vi "Thermopower-v2-SMU1norangespec.vi"(0 "Gate Start":dbl format="%#_13g", 1 "hold time (sec)":dbl=10.0 format="%#_13g", 2 "Gate step - extra milliseconds to wait":u32=20000, 4 "N Gate Intervals":i32=7, 5 "Gate Step":dbl=-6.0, 6 "N Heater Intervals":i32=7, 7 "Heater Step":dbl=3.3) -> ()   [LabVIEW 2016]
uses:
  <vilib>/Utility/file.llb/Write To Spreadsheet File (DBL).vi
  <vilib>/Utility/file.llb/Read From Spreadsheet File (DBL).vi
  Driver/New driver/Agilent 415X Series.lvlib
panel:
  out "Voltage across heater (VSU 1 and SMU4) 2":dbl[][](graph)
  out "error out 2":errorcluster
  out "Gate Voltage (SMU 3) 2":dbl[](graph)
  out "Thermal Voltage (SMU2), SMU1 is Common 2":dbl[](graph)
  out "SPA VISA resource name 2":refnum<visa-resource-name>
  out "Voltage across heater (VSU 1 and SMU4)":dbl[][](graph)
  out "Gate Voltage (SMU 3)":dbl[](graph)
  out "Thermal Voltage (SMU2), SMU1 is Common":dbl[](graph)
  in  "SPA VISA resource name":refnum<visa-resource-name>="GPIB0::14::INSTR"
  in  "error in (no error)":errorcluster
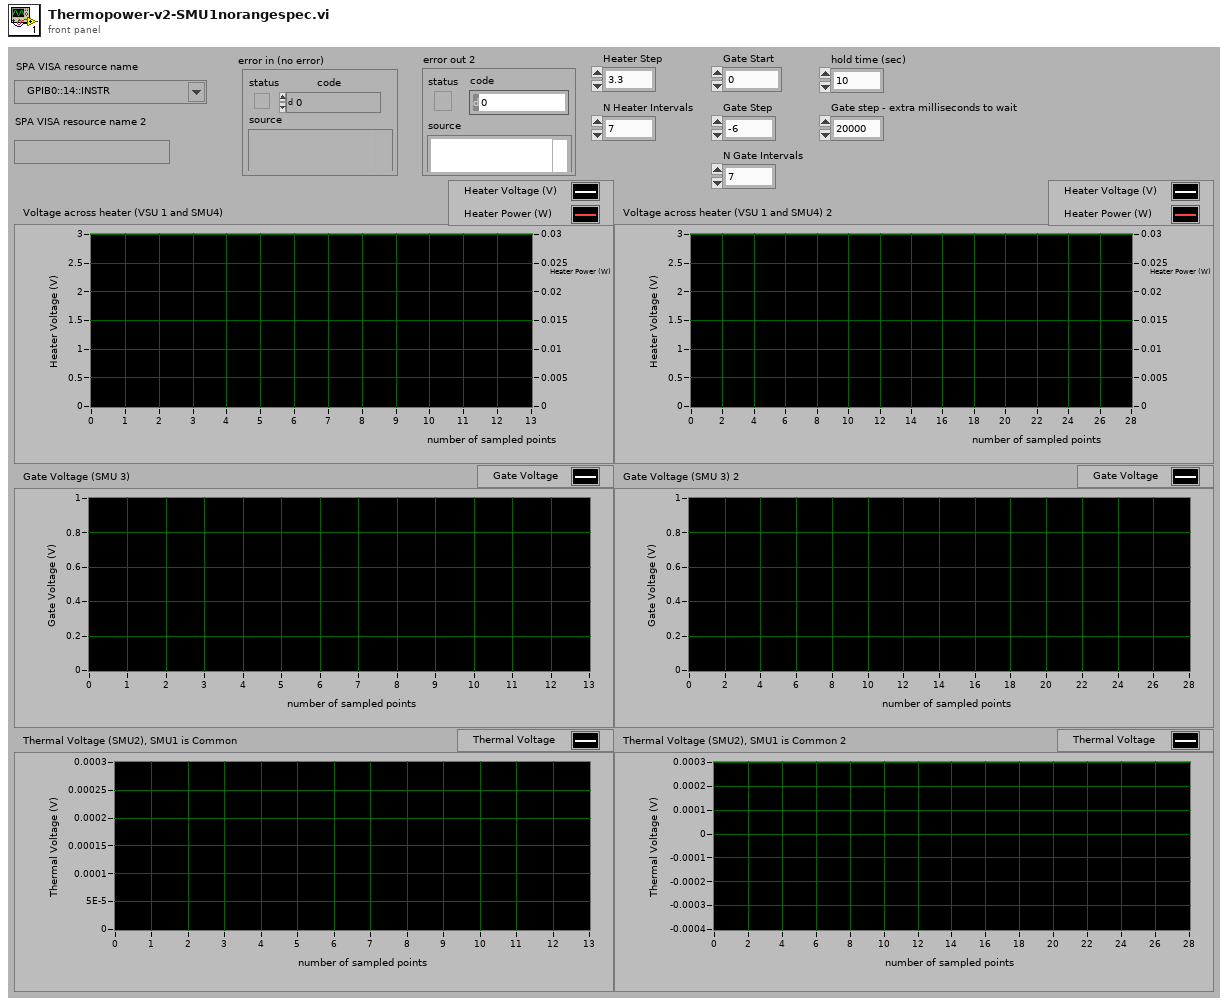
[diagram p1: front panel]
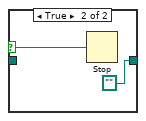
[diagram p3: hidden frame]
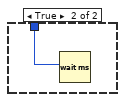
[diagram p4: hidden frame]
diagram:
  # "calculate end gate voltage"
  n1 = flat-sequence {
    tunnel: "error in (no error)" -> [w51]
    tunnel: "SPA VISA resource name" -> [w50]
    tunnel: [w49] -> w45
    tunnel: [w48] -> w44
    tunnel: w45 -> [w58]
    tunnel: w44 -> [w57]
    tunnel: [w54] -> w43
    tunnel: [w53] -> w42
    tunnel: w43 -> [w66]
    tunnel: w42 -> [w65]
    tunnel: [w64] -> w41
    tunnel: [w63] -> w40
    tunnel: w41 -> [w77]
    tunnel: w40 -> [w76]
    tunnel: [w75] -> w39
    tunnel: [w74] -> w38
    tunnel: w39 -> [w88]
    tunnel: w38 -> [w87]
    tunnel: [w86] -> w37
    tunnel: [w85] -> w35
    tunnel: w37 -> [w93]
    tunnel: [w94] -> w36
    tunnel: w35 -> [w92]
    tunnel: [w95] -> w34
    tunnel: w36 -> [w110]
    tunnel: w34 -> [w112]
    tunnel: [w111] -> w27
    tunnel: [w109] -> w26
    tunnel: w27 -> [w114]
    tunnel: w26 -> [w113]
    tunnel: [w117] -> w2
    tunnel: [w116] -> w1
    tunnel: [w127] -> w33
    tunnel: [w130] -> w32
    tunnel: [w129] -> w5
    tunnel: w2 -> [w127]
    tunnel: w1 -> [w128]
    frame #0 {
      n2 = call "Initialize.vi"("error in (no error)"=w51, "reset"=TRUE, "VISA resource name"=w50) -> ("error out"=w48:errorcluster, "VISA resource name out"=w49:refnum<visa-resource-name>)  [unwired: 2 in, 5 out]
    }
    frame #1 {
      n3 = call "Select-Meas. Mode.vi"("clear all channels"=TRUE, "error in (no error)"=w57, "measurement mode"=TRUE, "VISA resource name"=w58) -> ("error out"=w53:errorcluster, "VISA resource name out"=w54:refnum<visa-resource-name>)  [unwired: 1 in, 5 out]
    }
    frame #2 {
      w61 = 0 items=["0  ", "10K Ohms  ", "100K Ohms  ", "1M Ohms  "] ("series resistance *")
      w62 = 2 items=["V  ", "I  ", "  common  "] ("mode")
      w67 = 0 items=["SMU1  ", "SMU2  ", "SMU3  ", "SMU4  ", "SMU5  ", "SMU6  "] ("unit to configure")
      # "SMU1 configured to be common"
      n4 = call "Config-Chan-SMU-Sampling.vi"("VISA resource name in"=w66, "function"=TRUE, "series resistance *"=w61, "unit to configure"=w67, "V name (max 6 chars)"="Vgnd", "standby"=TRUE, "error in (no error)"=w65, "mode"=w62, "I name (max 6 chars)"="Ignd") -> ("VISA resource name out"=w64:refnum<visa-resource-name>, "error out"=w63:errorcluster)  [unwired: 5 out]
    }
    frame #3 {
      w71 = 0 items=["0  ", "10K Ohms  ", "100K Ohms  ", "1M Ohms  "] ("series resistance *")
      w73 = 1 items=["V  ", "I  ", "  common  "] ("mode")
      w78 = 1 items=["SMU1  ", "SMU2  ", "SMU3  ", "SMU4  ", "SMU5  ", "SMU6  "] ("unit to configure")
      # "SMU2 configured to source current (to be set to zero) \nand measure the thermal voltage"
      n5 = call "Config-Chan-SMU-Sampling.vi"("VISA resource name in"=w77, "function"=TRUE, "series resistance *"=w71, "unit to configure"=w78, "V name (max 6 chars)"="Vth", "standby"=TRUE, "error in (no error)"=w76, "mode"=w73, "I name (max 6 chars)"="Ith") -> ("VISA resource name out"=w75:refnum<visa-resource-name>, "error out"=w74:errorcluster)  [unwired: 5 out]
    }
    frame #4 {
      w82 = 0 items=["0  ", "10K Ohms  ", "100K Ohms  ", "1M Ohms  "] ("series resistance *")
      w84 = 0 items=["V  ", "I  ", "  common  "] ("mode")
      w89 = 2 items=["SMU1  ", "SMU2  ", "SMU3  ", "SMU4  ", "SMU5  ", "SMU6  "] ("unit to configure")
      # "SMU3 configured to source a gate voltage"
      n6 = call "Config-Chan-SMU-Sampling.vi"("VISA resource name in"=w88, "function"=TRUE, "series resistance *"=w82, "unit to configure"=w89, "V name (max 6 chars)"="Vg", "standby"=TRUE, "error in (no error)"=w87, "mode"=w84, "I name (max 6 chars)"="Ig") -> ("VISA resource name out"=w86:refnum<visa-resource-name>, "error out"=w85:errorcluster)  [unwired: 5 out]
    }
    frame #5 {
      w97 = 0 items=["0  ", "10K Ohms  ", "100K Ohms  ", "1M Ohms  "] ("series resistance *")
      w99 = 2 items=["V  ", "I  ", "  common  "] ("mode")
      w100 = 3 items=["SMU1  ", "SMU2  ", "SMU3  ", "SMU4  ", "SMU5  ", "SMU6  "] ("unit to configure")
      # "SMU4 configured to heater ground"
      n7 = call "Config-Chan-SMU-Sampling.vi"("VISA resource name in"=w93, "function"=TRUE, "series resistance *"=w97, "unit to configure"=w100, "V name (max 6 chars)"="Vhgnd", "standby"=TRUE, "error in (no error)"=w92, "mode"=w99, "I name (max 6 chars)"="Ihgnd") -> ("VISA resource name out"=w94:refnum<visa-resource-name>, "error out"=w95:errorcluster)  [unwired: 5 out]
    }
    frame #6 {
      # "VSU1 configured to source a voltage accross a heater"
      n8 = call "Config-Chan-VSUs-Sampling.vi"("VISA session"=w110, "VSU1 function"=TRUE, "VSU2 standby"=TRUE, "VSU1 standby"=FALSE, "VSU1 V name \n(max 6 chars)"="VSU1" ("V name (max 6 chars)"), "VSU2 V name \n(max 6 chars)"="VSU2" ("V name (max 6 chars)"), "error in (no error)"=w112, "VSU2 function"=FALSE) -> ("VISA resource name out"=w109:refnum<visa-resource-name>, "error out"=w111:errorcluster)  [unwired: 6 out]
    }
    frame #7 {
      n9 = VISA Write(VISA resource name=w113, write buffer=":PAGE:MEAS:MSET:SMU2:RANG:MODE FIX", error in (no error)=w114) -> (VISA resource name out=w126:refnum<visa-resource-name>, error out=w125:errorcluster)  [unwired: 1 out]
      n10 = VISA Write(VISA resource name=w126, write buffer=":PAGE:MEAS:MSET:SMU2:RANG 2", error in (no error)=w125) -> (VISA resource name out=w121:refnum<visa-resource-name>, error out=w120:errorcluster)  [unwired: 1 out]
      n11 = VISA Write(VISA resource name=w121, write buffer=":PAGE:MEAS:MSET:ITIM LONG", error in (no error)=w120) -> (VISA resource name out=w119:refnum<visa-resource-name>, error out=w118:errorcluster)  [unwired: 1 out]
      n12 = VISA Write(VISA resource name=w119, write buffer=":PAGE:MEAS:MSET:ITIM:LONG 10", error in (no error)=w118) -> (VISA resource name out=w117:refnum<visa-resource-name>, error out=w116:errorcluster)  [unwired: 1 out]
    }
    frame #8 {
      w129 = 0.0 ("source (V or A)")
      w131 = u16 1 items=["SMU 1", "SMU2", "SMU3", "SMU4", "SMU5", "SMU6", "VSU1", "VSU2"] ("unit (SMU1:0)")
      n13 = call "Config-Sampling-Const-Source.vi"("compliance (SMUs only)"=0.0001, "error in (no error)"=w128, "source (V or A)"=w129, "unit (SMU1:0)"=w131, "VISA session"=w127) -> ("error out"=w130:errorcluster)  [unwired: 6 out]
    }
  }
  n14 = Subtract(x="N Gate Intervals", y=1) -> (x-y=w13:i32)
  n15 = Multiply(x=w13, y="Gate Step") -> (x*y=w11:dbl)
  n16 = Add(x=w11, y="Gate Start") -> (x+y=w10:dbl)
  n17 = call "File Dialog"("start path"=path "C:/users old/khk30", "pattern (all files)"="*.txt") -> ("selected path"=w30:path, "cancelled"=w29:bool)  [unwired: 10 in, 2 out]
  n18 = case shown="False" w29 {
    selector: w29 -> [_ w135]
    tunnel: w30 -> [w133 _]
    tunnel: [w133 path ""] -> w17
    frame False {
    }
    frame True {
      n19 = Stop(stop? (T)=w135) -> ()
    }
  }
  n20 = for {
    N: "N Gate Intervals" -> [_]
    tunnel: w17 -> [w147]
    tunnel: w33 -> [w146]
    tunnel: w32 -> [w145]
    tunnel: [w143] -> w21
    tunnel: [w142] -> w20
    tunnel: "N Heater Intervals" -> [w141]
    tunnel: "Gate Step" -> [w140]
    tunnel: "Gate Start" -> [w139]
    tunnel: "Heater Step" -> [w138]
    tunnel: "Gate step - extra milliseconds to wait" -> [w137]
    tunnel: [w136] -> w6 mode=indexing
    i -> [w144]
    n21 = flat-sequence {
      tunnel: w144 -> [w299]
      tunnel: [w304] -> w149
      tunnel: [w303] -> w148
      tunnel: w146 -> [w302]
      tunnel: w145 -> [w301]
      tunnel: w140 -> [w296]
      tunnel: w139 -> [w295]
      frame #0 {
        w305 = u16 2 items=["SMU 1", "SMU2", "SMU3", "SMU4", "SMU5", "SMU6", "VSU1", "VSU2"] ("unit (SMU1:0)")
        n22 = Multiply(x=w296, y=w299) -> (x*y=w298:dbl)
        n23 = Add(x=w295, y=w298) -> (x+y=w297:dbl)
        n24 = call "Config-Sampling-Const-Source.vi"("compliance (SMUs only)"=0.001, "error in (no error)"=w301, "source (V or A)"=w297, "unit (SMU1:0)"=w305, "VISA session"=w302) -> ("error out"=w303:errorcluster, "VISA resource name out"=w304:refnum<visa-resource-name>)  [unwired: 5 out]
      }
    }
    n25 = for {
      N: w141 -> [_]
      tunnel: w149 -> [w168]
      tunnel: w148 -> [w167]
      tunnel: w147 -> [w166]
      tunnel: w144 -> [w159]
      tunnel: [w154] -> w143
      tunnel: [w153] -> w142
      tunnel: w138 -> [w152]
      tunnel: w137 -> [w151]
      tunnel: [w150] -> w136 mode=indexing
      i -> [w169]
      n26 = flat-sequence {
        tunnel: [w186] -> w179
        tunnel: [w185] -> w178
        tunnel: w169 -> [w181]
        tunnel: w168 -> [w184]
        tunnel: w167 -> [w183]
        tunnel: [w181] -> w160
        tunnel: w152 -> [w180]
        tunnel: w179 -> [w196]
        tunnel: w178 -> [w194]
        tunnel: [w195] -> w177
        tunnel: [w194] -> w176
        tunnel: w160 -> [w190]
        tunnel: w159 -> [w189]
        tunnel: w151 -> [w188]
        tunnel: w177 -> [w203]
        tunnel: w176 -> [w202]
        tunnel: [w201] -> w175
        tunnel: [w200] -> w174
        tunnel: ["hold time (sec)"] -> w150
        tunnel: w175 -> [w213]
        tunnel: w174 -> [w212]
        tunnel: [w211] -> w173
        tunnel: [w210] -> w172
        tunnel: w173 -> [w219]
        tunnel: w172 -> [w218]
        tunnel: [w217] -> w171
        tunnel: [w216] -> w170
        tunnel: w171 -> [w238]
        tunnel: w170 -> [w237]
        tunnel: w166 -> [w239]
        tunnel: [w239] -> w165
        tunnel: [w239] -> w164
        tunnel: [w225] -> w162
        tunnel: [w227] -> w154
        tunnel: w165 -> [w266]
        tunnel: [w264] -> w158
        tunnel: w164 -> [w264]
        tunnel: w162 -> [w261]
        tunnel: [w261] -> w156
        tunnel: w158 -> [w270]
        tunnel: [w270] -> w157
        tunnel: w156 -> [w271]
        tunnel: [w271] -> w155
        tunnel: w157 -> [w276]
        tunnel: [w276] -> w163
        tunnel: w155 -> [w272]
        tunnel: [w272] -> w161
        tunnel: w163 -> [w290]
        tunnel: w161 -> [w281]
        tunnel: [w281] -> w153
        frame #0 {
          w187 = u16 6 items=["SMU 1", "SMU2", "SMU3", "SMU4", "SMU5", "SMU6", "VSU1", "VSU2"] ("unit (SMU1:0)")
          n27 = Multiply(x=w180, y=w181) -> (x*y=w182:dbl)
          n28 = call "Config-Sampling-Const-Source.vi"("error in (no error)"=w183, "source (V or A)"=w182, "unit (SMU1:0)"=w187, "VISA session"=w184) -> ("error out"=w186:errorcluster, "VISA resource name out"=w185:refnum<visa-resource-name>)  [unwired: 1 in, 5 out]
        }
        frame #1 {
          n29 = Equal To 0?(x=w190) -> (x = 0?=w191:bool)
          n30 = Greater Than 0?(x=w189) -> (x > 0?=w192:bool)
          n31 = And(x=w191, y=w192) -> (x .and. y?=w193:bool)
          n32 = call "Config-Display-List.vi"("error in (no error)"=w196, "list (max 8 elements)"=string[] ["Vth", "Ith", "VSU1", "Ihgnd", "Vg", "Ig", "Ignd"], "VISA session"=w194) -> ("error out"=w195:errorcluster)  [unwired: 1 in, 7 out]
          n33 = case shown="False" w193 {
            tunnel: w188 -> [_ w198]
            frame False {
            }
            frame True {
              n34 = Wait (ms)(milliseconds to wait=w198) -> ()  [unwired: 1 out]
            }
          }
        }
        frame #2 {
          w204 = 100.0  # sampling time limit
          w205 = 0 items=["linear", "log 10", "log 25", "log 50", "thinned out"] ("mode (linear: 0)")
          w206 = 0 items=["auto (linear only)", "no limit", "set limit "] ("sampling time\n(linear/thinned-out only)")
          w207 = 0.1  # initial interval (sec)
          w208 = 10  # num. of events
          w209 = 1  # number of samples
          n35 = call "Config-Sampling-Parameters.vi"("VISA session"=w202, "mode (linear: 0)"=w205, "initial interval (sec)"=w207, "sampling time\n(linear/thinned-out only)"=w206, "number of samples"=w209, "error in (no error)"=w203, "sampling time limit"=w204, "num. of events"=w208, "hold time (sec)"="hold time (sec)") -> ("VISA resource name out"=w200:refnum<visa-resource-name>, "error out"=w201:errorcluster)  [unwired: 7 in, 10 out]
        }
        frame #3 {
          w215 = 2 items=["short  ", "medium  ", "long  "] ("integration time")
          n36 = call "Config-Meas-Timing.vi"("# PLCs for long integration time"=1, "error in (no error)"=w213, "integration time"=w215, "VISA session"=w212) -> ("error out"=w211:errorcluster, "VISA resource name out"=w210:refnum<visa-resource-name>)  [unwired: 2 in, 4 out]
        }
        frame #4 {
          w221 = 1 items=["stop  ", "single  ", "single-append  ", "stress start  ", "continuous  ", "standby on  ", "standby off  ", "zero  "] ("function (stop:0)")
          n37 = call "Op-Start-Stop.vi"("time to wait (30000ms)"=600000, "error in (no error)"=w219, "function (stop:0)"=w221, "wait until finish"=TRUE, "VISA resource name"=w218) -> ("error out"=w217:errorcluster, "VISA resource name out"=w216:refnum<visa-resource-name>)  [unwired: 5 out]
        }
        frame #5 {
          # "Computes Heater power via P=VI"
          n38 = call "4155C DOWNLOAD variable.vi"("error in (no error)"=w238, "Variable name"="Vth", "VISA resource name in"=w237) -> ("error out"=w246:errorcluster, "Output data"=w233:dbl[], "VISA Resource Name out"=w251:refnum<visa-resource-name>)  [unwired: 2 out]
          n39 = call "4155C DOWNLOAD variable.vi"("error in (no error)"=w246, "Variable name"="Ith", "VISA resource name in"=w251) -> ("error out"=w245:errorcluster, "Output data"=w234:dbl[], "VISA Resource Name out"=w250:refnum<visa-resource-name>)  [unwired: 2 out]
          n40 = call "4155C DOWNLOAD variable.vi"("error in (no error)"=w245, "Variable name"="VSU1", "VISA resource name in"=w250) -> ("error out"=w244:errorcluster, "Output data"=w231:dbl[], "VISA Resource Name out"=w249:refnum<visa-resource-name>)  [unwired: 2 out]
          n41 = call "4155C DOWNLOAD variable.vi"("error in (no error)"=w244, "Variable name"="Ihgnd", "VISA resource name in"=w249) -> ("error out"=w243:errorcluster, "Output data"=w232:dbl[], "VISA Resource Name out"=w248:refnum<visa-resource-name>)  [unwired: 2 out]
          n42 = Multiply(x=w231, y=w232) -> (x*y=w236:dbl[])
          n43 = Absolute Value(x=w236) -> (abs(x)=w230:dbl[])
          n44 = call "4155C DOWNLOAD variable.vi"("error in (no error)"=w243, "Variable name"="Vg", "VISA resource name in"=w248) -> ("error out"=w242:errorcluster, "Output data"=w235:dbl[], "VISA Resource Name out"=w247:refnum<visa-resource-name>)  [unwired: 2 out]
          n45 = call "4155C DOWNLOAD variable.vi"("error in (no error)"=w242, "Variable name"="Ig", "VISA resource name in"=w247) -> ("error out"=w226:errorcluster, "Output data"=w224:dbl[], "VISA Resource Name out"=w229:refnum<visa-resource-name>)  [unwired: 2 out]
          n46 = call "4155C DOWNLOAD variable.vi"("error in (no error)"=w226, "Variable name"="Ignd", "VISA resource name in"=w229) -> ("error out"=w225:errorcluster, "Output data"=w223:dbl[], "VISA Resource Name out"=w227:refnum<visa-resource-name>)  [unwired: 2 out]
          n47 = Build Array(w230, w231, w232, w233, w234, w235, w224, w223) -> (w241:dbl[][])
          n48 = call-poly <vilib>:"Write To Spreadsheet File.vi"("transpose? (no:F)"=TRUE, "format (%.3f)"="%.13f", "append to file? (new file:F)"=TRUE, "2D data"=w241, "file path (dialog if empty)"=w239) -> ()  [unwired: 1 in, 3 out]
        }
        frame #6 {
          # "plot the thermal voltage after reading the file"
          n49 = call-poly <vilib>:"Read From Spreadsheet File.vi"("transpose (no:F)"=TRUE, "format (%.3f)"="%.13f", "max characters/row  (no limit:0)"=0, "number of rows (all:-1)"=-1, "file path (dialog if empty)"=w266) -> ("all rows"=w263:dbl[][])  [unwired: 6 out]
          n50 = Index Array(array=w263, index (row)=3) -> (element=→"Thermal Voltage (SMU2), SMU1 is Common":dbl[])  [unwired: 1 in]
        }
        frame #7 {
        }
        frame #8 {
          # "plot the gate voltage after reading the file"
          n51 = call-poly <vilib>:"Read From Spreadsheet File.vi"("transpose (no:F)"=TRUE, "format (%.3f)"="%.13f", "max characters/row  (no limit:0)"=0, "number of rows (all:-1)"=-1, "file path (dialog if empty)"=w276) -> ("all rows"=w275:dbl[][])  [unwired: 6 out]
          n52 = Index Array(array=w275, index (row)=5) -> (element=→"Gate Voltage (SMU 3)":dbl[])  [unwired: 1 in]
        }
        frame #9 {
          # "plot the voltage across the heater and the \npower dissipated by the heater after reading the file"
          n53 = call-poly <vilib>:"Read From Spreadsheet File.vi"("transpose (no:F)"=TRUE, "format (%.3f)"="%.13f", "max characters/row  (no limit:0)"=0, "number of rows (all:-1)"=-1, "file path (dialog if empty)"=w290) -> ("all rows"=w288:dbl[][])  [unwired: 6 out]
          n54 = Index Array(array=w288, index (row)=1) -> (element=w282:dbl[])  [unwired: 1 in]
          n55 = Index Array(array=w288, index (row)=2) -> (element=w286:dbl[])  [unwired: 1 in]
          n56 = Multiply(x=w282, y=w286) -> (x*y=w285:dbl[])
          n57 = Absolute Value(x=w285) -> (abs(x)=w284:dbl[])
          n58 = Build Array(w282, w284) -> (→"Voltage across heater (VSU 1 and SMU4)":dbl[][])
        }
      }
    }
  }
  n59 = flat-sequence {
    tunnel: [w313] -> w25
    tunnel: [w312] -> w24
    tunnel: w21 -> [w307]
    tunnel: w20 -> [w306]
    tunnel: w25 -> [w324]
    tunnel: w24 -> [w323]
    tunnel: [w318] -> w4
    tunnel: [w317] -> w3
    tunnel: [w328] -> w23
    tunnel: [w329] -> w22
    tunnel: w4 -> [w331]
    tunnel: w3 -> [w330]
    tunnel: w23 -> [w339]
    tunnel: w22 -> [w340]
    tunnel: [w338] -> w18
    tunnel: [w337] -> w19
    tunnel: w5 -> [w336]
    frame #0 {
      w310 = 0 items=["0  ", "10K Ohms  ", "100K Ohms  ", "1M Ohms  "] ("series resistance *")
      w311 = 2 items=["V  ", "I  ", "  common  "] ("mode")
      w314 = 1 items=["SMU1  ", "SMU2  ", "SMU3  ", "SMU4  ", "SMU5  ", "SMU6  "] ("unit to configure")
      # "SMU2 configured to be common"
      n60 = call "Config-Chan-SMU-Sampling.vi"("VISA resource name in"=w307, "function"=TRUE, "series resistance *"=w310, "unit to configure"=w314, "V name (max 6 chars)"="Vgnd", "standby"=TRUE, "error in (no error)"=w306, "mode"=w311, "I name (max 6 chars)"="Ignd") -> ("VISA resource name out"=w313:refnum<visa-resource-name>, "error out"=w312:errorcluster)  [unwired: 5 out]
    }
    frame #1 {
      w320 = 0 items=["0  ", "10K Ohms  ", "100K Ohms  ", "1M Ohms  "] ("series resistance *")
      w322 = 1 items=["V  ", "I  ", "  common  "] ("mode")
      w325 = 0 items=["SMU1  ", "SMU2  ", "SMU3  ", "SMU4  ", "SMU5  ", "SMU6  "] ("unit to configure")
      # "SMU2 configured to source current (to be set to zero) \nand measure the thermal voltage"
      n61 = call "Config-Chan-SMU-Sampling.vi"("VISA resource name in"=w324, "function"=TRUE, "series resistance *"=w320, "unit to configure"=w325, "V name (max 6 chars)"="Vth", "standby"=TRUE, "error in (no error)"=w323, "mode"=w322, "I name (max 6 chars)"="Ith") -> ("VISA resource name out"=w318:refnum<visa-resource-name>, "error out"=w317:errorcluster)  [unwired: 5 out]
    }
    frame #2 {
      n62 = VISA Write(VISA resource name=w331, write buffer=":PAGE:MEAS:MSET:SMU1:RANG:MODE FIX", error in (no error)=w330) -> (VISA resource name out=w334:refnum<visa-resource-name>, error out=w333:errorcluster)  [unwired: 1 out]
      n63 = VISA Write(VISA resource name=w334, write buffer=":PAGE:MEAS:MSET:SMU1:RANG 2", error in (no error)=w333) -> (VISA resource name out=w329:refnum<visa-resource-name>, error out=w328:errorcluster)  [unwired: 1 out]
    }
    frame #3 {
      w341 = u16 0 items=["SMU 1", "SMU2", "SMU3", "SMU4", "SMU5", "SMU6", "VSU1", "VSU2"] ("unit (SMU1:0)")
      n64 = call "Config-Sampling-Const-Source.vi"("compliance (SMUs only)"=0.0001, "error in (no error)"=w339, "source (V or A)"=w336, "unit (SMU1:0)"=w341, "VISA session"=w340) -> ("error out"=w337:errorcluster, "VISA resource name out"=w338:refnum<visa-resource-name>)  [unwired: 5 out]
    }
  }
  n65 = for {
    N: "N Gate Intervals" -> [_]
    tunnel: w17 -> [w354]
    tunnel: w18 -> [w353]
    tunnel: w19 -> [w352]
    tunnel: [w350] -> _
    tunnel: [w349] -> _
    tunnel: "N Heater Intervals" -> [w348]
    tunnel: w10 -> [w347]
    tunnel: "Gate Step" -> [w346]
    tunnel: "Heater Step" -> [w345]
    tunnel: "Gate step - extra milliseconds to wait" -> [w344]
    tunnel: w6 -> [w343] mode=indexing
    i -> [w351]
    n66 = flat-sequence {
      tunnel: w351 -> [w511]
      tunnel: [w516] -> w356
      tunnel: [w515] -> w355
      tunnel: w353 -> [w514]
      tunnel: w352 -> [w513]
      tunnel: w347 -> [w509]
      tunnel: w346 -> [w507]
      frame #0 {
        w517 = u16 2 items=["SMU 1", "SMU2", "SMU3", "SMU4", "SMU5", "SMU6", "VSU1", "VSU2"] ("unit (SMU1:0)")
        n67 = Multiply(x=w507, y=w511) -> (x*y=w508:dbl)
        n68 = Subtract(x=w509, y=w508) -> (x-y=w510:dbl)
        n69 = call "Config-Sampling-Const-Source.vi"("compliance (SMUs only)"=0.001, "error in (no error)"=w513, "source (V or A)"=w510, "unit (SMU1:0)"=w517, "VISA session"=w514) -> ("error out"=w515:errorcluster, "VISA resource name out"=w516:refnum<visa-resource-name>)  [unwired: 5 out]
      }
    }
    n70 = for {
      N: w348 -> [_]
      tunnel: w356 -> [w375]
      tunnel: w355 -> [w374]
      tunnel: w354 -> [w373]
      tunnel: w351 -> [w366]
      tunnel: [w361] -> w350
      tunnel: [w360] -> w349
      tunnel: w345 -> [w359]
      tunnel: w344 -> [w358]
      tunnel: w343 -> [w357] mode=indexing
      i -> [w376]
      n71 = flat-sequence {
        tunnel: [w393] -> w386
        tunnel: [w392] -> w385
        tunnel: w376 -> [w388]
        tunnel: w375 -> [w391]
        tunnel: w374 -> [w390]
        tunnel: [w388] -> w367
        tunnel: w359 -> [w387]
        tunnel: w386 -> [w403]
        tunnel: w385 -> [w401]
        tunnel: [w402] -> w384
        tunnel: [w401] -> w383
        tunnel: w367 -> [w397]
        tunnel: w366 -> [w396]
        tunnel: w358 -> [w395]
        tunnel: w384 -> [w410]
        tunnel: w383 -> [w409]
        tunnel: [w408] -> w382
        tunnel: [w407] -> w381
        tunnel: w357 -> [w406]
        tunnel: w382 -> [w420]
        tunnel: w381 -> [w419]
        tunnel: [w418] -> w380
        tunnel: [w417] -> w379
        tunnel: w380 -> [w426]
        tunnel: w379 -> [w425]
        tunnel: [w424] -> w378
        tunnel: [w423] -> w377
        tunnel: w378 -> [w445]
        tunnel: w377 -> [w444]
        tunnel: w373 -> [w446]
        tunnel: [w446] -> w372
        tunnel: [w446] -> w371
        tunnel: [w433] -> w369
        tunnel: [w432] -> w361
        tunnel: w372 -> [w473]
        tunnel: [w471] -> w365
        tunnel: w371 -> [w471]
        tunnel: w369 -> [w468]
        tunnel: [w468] -> w363
        tunnel: w365 -> [w477]
        tunnel: [w477] -> w364
        tunnel: w363 -> [w478]
        tunnel: [w478] -> w362
        tunnel: w364 -> [w483]
        tunnel: [w483] -> w370
        tunnel: w362 -> [w479]
        tunnel: [w479] -> w368
        tunnel: w370 -> [w502]
        tunnel: w368 -> [w488]
        tunnel: [w488] -> w360
        frame #0 {
          w394 = u16 6 items=["SMU 1", "SMU2", "SMU3", "SMU4", "SMU5", "SMU6", "VSU1", "VSU2"] ("unit (SMU1:0)")
          n72 = Multiply(x=w387, y=w388) -> (x*y=w389:dbl)
          n73 = call "Config-Sampling-Const-Source.vi"("error in (no error)"=w390, "source (V or A)"=w389, "unit (SMU1:0)"=w394, "VISA session"=w391) -> ("error out"=w393:errorcluster, "VISA resource name out"=w392:refnum<visa-resource-name>)  [unwired: 1 in, 5 out]
        }
        frame #1 {
          n74 = Equal To 0?(x=w397) -> (x = 0?=w398:bool)
          n75 = Greater Than 0?(x=w396) -> (x > 0?=w399:bool)
          n76 = And(x=w398, y=w399) -> (x .and. y?=w400:bool)
          n77 = call "Config-Display-List.vi"("error in (no error)"=w403, "list (max 8 elements)"=string[] ["Vth", "Ith", "VSU1", "Ihgnd", "Vg", "Ig", "Ignd"], "VISA session"=w401) -> ("error out"=w402:errorcluster)  [unwired: 1 in, 7 out]
          n78 = case shown="True" w400 {
            tunnel: w395 -> [_ w405]
            frame False {
            }
            frame True {
              n79 = Wait (ms)(milliseconds to wait=w405) -> ()  [unwired: 1 out]
            }
          }
        }
        frame #2 {
          w411 = 100.0  # sampling time limit
          w412 = 0 items=["linear", "log 10", "log 25", "log 50", "thinned out"] ("mode (linear: 0)")
          w413 = 0 items=["auto (linear only)", "no limit", "set limit "] ("sampling time\n(linear/thinned-out only)")
          w414 = 0.1  # initial interval (sec)
          w415 = 10  # num. of events
          w416 = 1  # number of samples
          n80 = call "Config-Sampling-Parameters.vi"("VISA session"=w409, "mode (linear: 0)"=w412, "initial interval (sec)"=w414, "sampling time\n(linear/thinned-out only)"=w413, "number of samples"=w416, "error in (no error)"=w410, "sampling time limit"=w411, "num. of events"=w415, "hold time (sec)"=w406) -> ("VISA resource name out"=w407:refnum<visa-resource-name>, "error out"=w408:errorcluster)  [unwired: 7 in, 10 out]
        }
        frame #3 {
          w422 = 2 items=["short  ", "medium  ", "long  "] ("integration time")
          n81 = call "Config-Meas-Timing.vi"("# PLCs for long integration time"=1, "error in (no error)"=w420, "integration time"=w422, "VISA session"=w419) -> ("error out"=w418:errorcluster, "VISA resource name out"=w417:refnum<visa-resource-name>)  [unwired: 2 in, 4 out]
        }
        frame #4 {
          w428 = 1 items=["stop  ", "single  ", "single-append  ", "stress start  ", "continuous  ", "standby on  ", "standby off  ", "zero  "] ("function (stop:0)")
          n82 = call "Op-Start-Stop.vi"("time to wait (30000ms)"=600000, "error in (no error)"=w426, "function (stop:0)"=w428, "wait until finish"=TRUE, "VISA resource name"=w425) -> ("error out"=w424:errorcluster, "VISA resource name out"=w423:refnum<visa-resource-name>)  [unwired: 5 out]
        }
        frame #5 {
          # "Computes Heater power via P=VI"
          n83 = call "4155C DOWNLOAD variable.vi"("error in (no error)"=w445, "Variable name"="Vth", "VISA resource name in"=w444) -> ("error out"=w453:errorcluster, "Output data"=w439:dbl[], "VISA Resource Name out"=w458:refnum<visa-resource-name>)  [unwired: 2 out]
          n84 = call "4155C DOWNLOAD variable.vi"("error in (no error)"=w453, "Variable name"="Ith", "VISA resource name in"=w458) -> ("error out"=w452:errorcluster, "Output data"=w440:dbl[], "VISA Resource Name out"=w457:refnum<visa-resource-name>)  [unwired: 2 out]
          n85 = call "4155C DOWNLOAD variable.vi"("error in (no error)"=w452, "Variable name"="VSU1", "VISA resource name in"=w457) -> ("error out"=w451:errorcluster, "Output data"=w437:dbl[], "VISA Resource Name out"=w456:refnum<visa-resource-name>)  [unwired: 2 out]
          n86 = call "4155C DOWNLOAD variable.vi"("error in (no error)"=w451, "Variable name"="Ihgnd", "VISA resource name in"=w456) -> ("error out"=w450:errorcluster, "Output data"=w438:dbl[], "VISA Resource Name out"=w455:refnum<visa-resource-name>)  [unwired: 2 out]
          n87 = Multiply(x=w437, y=w438) -> (x*y=w443:dbl[])
          n88 = Absolute Value(x=w443) -> (abs(x)=w436:dbl[])
          n89 = call "4155C DOWNLOAD variable.vi"("error in (no error)"=w450, "Variable name"="Vg", "VISA resource name in"=w455) -> ("error out"=w449:errorcluster, "Output data"=w441:dbl[], "VISA Resource Name out"=w454:refnum<visa-resource-name>)  [unwired: 2 out]
          n90 = call "4155C DOWNLOAD variable.vi"("error in (no error)"=w449, "Variable name"="Ig", "VISA resource name in"=w454) -> ("error out"=w434:errorcluster, "Output data"=w442:dbl[], "VISA Resource Name out"=w435:refnum<visa-resource-name>)  [unwired: 2 out]
          n91 = call "4155C DOWNLOAD variable.vi"("error in (no error)"=w434, "Variable name"="Ignd", "VISA resource name in"=w435) -> ("error out"=w433:errorcluster, "Output data"=w431:dbl[], "VISA Resource Name out"=w432:refnum<visa-resource-name>)  [unwired: 2 out]
          "SPA VISA resource name 2" <- w432
          n92 = Build Array(w436, w437, w438, w439, w440, w441, w442, w431) -> (w448:dbl[][])
          n93 = call-poly <vilib>:"Write To Spreadsheet File.vi"("transpose? (no:F)"=TRUE, "format (%.3f)"="%.13f", "append to file? (new file:F)"=TRUE, "2D data"=w448, "file path (dialog if empty)"=w446) -> ()  [unwired: 1 in, 3 out]
        }
        frame #6 {
          # "plot the thermal voltage after reading the file"
          n94 = call-poly <vilib>:"Read From Spreadsheet File.vi"("transpose (no:F)"=TRUE, "format (%.3f)"="%.13f", "max characters/row  (no limit:0)"=0, "number of rows (all:-1)"=-1, "file path (dialog if empty)"=w473) -> ("all rows"=w470:dbl[][])  [unwired: 6 out]
          n95 = Index Array(array=w470, index (row)=3) -> (element=→"Thermal Voltage (SMU2), SMU1 is Common 2":dbl[])  [unwired: 1 in]
        }
        frame #7 {
        }
        frame #8 {
          # "plot the gate voltage after reading the file"
          n96 = call-poly <vilib>:"Read From Spreadsheet File.vi"("transpose (no:F)"=TRUE, "format (%.3f)"="%.13f", "max characters/row  (no limit:0)"=0, "number of rows (all:-1)"=-1, "file path (dialog if empty)"=w483) -> ("all rows"=w482:dbl[][])  [unwired: 6 out]
          n97 = Index Array(array=w482, index (row)=5) -> (element=→"Gate Voltage (SMU 3) 2":dbl[])  [unwired: 1 in]
        }
        frame #9 {
          # "plot the voltage across the heater and the \npower dissipated by the heater after reading the file"
          n98 = call-poly <vilib>:"Read From Spreadsheet File.vi"("transpose (no:F)"=TRUE, "format (%.3f)"="%.13f", "max characters/row  (no limit:0)"=0, "number of rows (all:-1)"=-1, "file path (dialog if empty)"=w502) -> ("all rows"=w500:dbl[][])  [unwired: 6 out]
          n99 = Index Array(array=w500, index (row)=1) -> (element=w494:dbl[])  [unwired: 1 in]
          n100 = Index Array(array=w500, index (row)=2) -> (element=w498:dbl[])  [unwired: 1 in]
          n101 = property on="Voltage across heater (VSU 1 and SMU4) 2" class="WFGraph (strict)"(error in=w488, "Active Plot"=u32 0, "Plot.YScaleIdx"=u32 0 ("Plot.Y Scale Index"), "Active Plot"=u32 1, "Plot.YScaleIdx"=u32 1 ("Plot.Y Scale Index")) -> (error out=→"error out 2":errorcluster)  [unwired: 1 in, 1 out]
          n102 = Multiply(x=w494, y=w498) -> (x*y=w497:dbl[])
          n103 = Absolute Value(x=w497) -> (abs(x)=w496:dbl[])
          n104 = Build Array(w494, w496) -> (→"Voltage across heater (VSU 1 and SMU4) 2":dbl[][])
        }
      }
    }
  }
